vi "Initialize From Settings.vi"(8 "error in (no error)":errorcluster, 10 "settings":cluster{"key":string, "value":string}[](array[cluster]), 11 "Core Channels Configuration in":refnum<class "Channel Configuration.lvclass">) -> (0 "error out":errorcluster, 3 "Core Channels Configuration out":refnum<class "Channel Configuration.lvclass">)   [LabVIEW 2017, in "DSF Core.lvlib" / "Channel Configuration.lvclass"]
uses:
  Channel Configuration.lvclass
  Channel Configuration.lvclass/Channel Configuration.ctl
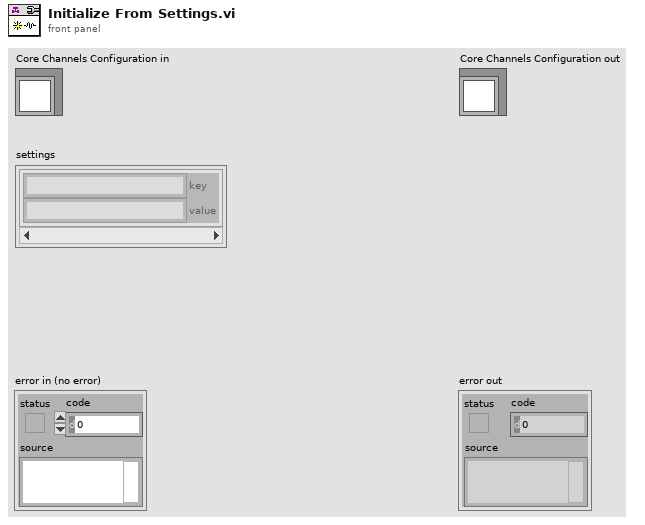
[diagram p1: front panel]
types:
  T1 = cluster{"name":string, "units":string, "engine data type":enum8{"Bool", "SGL", "DBL", "I8", "I16", "I32", "I64", "U8", "U16", "U32", "U64"}, "string data type":enum8{"Bool", "SGL", "DBL", "I8", "I16", "I32", "I64", "U8", "U16", "U32", "U64"}, "string offset":u64}
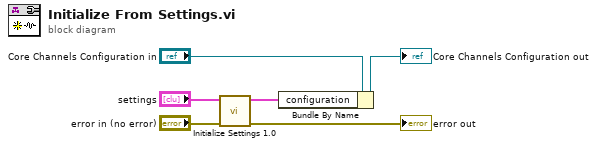
[diagram p0: block diagram]
diagram:
  n1 = call "Initialize Settings 1.0.vi"("error in (no error)"="error in (no error)", "settings 1.0"="settings") -> ("error out"=→"error out":errorcluster, "configuration 1.0"=w1:T1)  [unwired: 8 in]
  n2 = Bundle By Name(cluster="Core Channels Configuration in", "configuration"=w1) -> (→"Core Channels Configuration out":refnum<class "Channel Configuration.lvclass">)
